vi "FlatToRichnixnet_grpc_DbAddAlias64Request.vi"(5 "OutputClusterType":T1, 11 "InputCluster":T2) -> (3 "OutputCluster":T1)   [LabVIEW 2025, in "xnet-grpc_client.lvlib"]
uses:
  nixnet_grpc_DbAddAlias64Request_Flat.ctl
  nixnet_grpc_DbAddAlias64Request.ctl
  xnet-grpc_client.lvlib
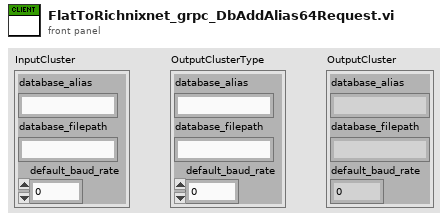
[diagram p1: front panel]
types:
  T1 = typedef "xnet-grpc_client.lvlib/nixnet_grpc_DbAddAlias64Request.ctl" = cluster{"database_alias":string, "database_filepath":string, "default_baud_rate":u64}
  T2 = typedef "xnet-grpc_client.lvlib/nixnet_grpc_DbAddAlias64Request_Flat.ctl" = cluster{"database_alias":string, "database_filepath":string, "default_baud_rate":u64}
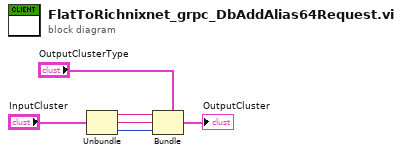
[diagram p0: block diagram]
diagram:
  n1 = Unbundle "Unbundle"("InputCluster") -> ("database_alias"=w3:string, "database_filepath"=w2:string, "default_baud_rate"=w1:u64)
  n2 = Bundle "Bundle"(cluster="OutputClusterType", "database_alias"=w3, "database_filepath"=w2, "default_baud_rate"=w1) -> (→"OutputCluster":T1)
